vi "Open Utility Motors.vi"(9 "CAN IDs":u8[](array[numeric])=[0, 0, 0, 0, 0, 0, 0]) -> ()   [LabVIEW 2018]
uses:
  <vilib>/Rock Robotics/WPI/ThirdParty/Phoenix-LabVIEW/Motor Controller/Controls/CTRE_Phoenix_MotorControl_NeutralMode.ctl
  <vilib>/Rock Robotics/WPI/Switch/WPI_SwitchOpenLimit.vi
  <vilib>/Rock Robotics/SystemInterfaces/DIO/FPGA_DIOChannel.ctl
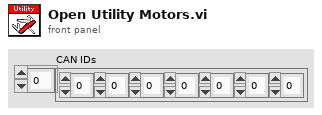
[diagram p1: front panel]
types:
  T1 = typedef "CTRE_Phoenix_MotorControl_NeutralMode.ctl" = enum8{"EEPROMSetting", "Override to Coast", "Override to Brake"}
  T2 = typedef "WPI_MotorControlDeviceRef.ctl" = cluster{"DeviceStatus":errorcluster, "Type":T3, "PWM":cluster{"PWM Channel":T4, "DeadBand":T5}, "CAN":cluster{"Device Number":u8, "SetOutput VI Ref":variant, "GetOutput VI Ref":variant, "Enable VI Ref":variant, "Disable VI Ref":variant, "Data":variant}, "Invert":bool, "DIO PWM":cluster{"PWM \"Enable\" Channel":T4, "DIOChannel":T6, "PWM Rate":dbl}}
  T3 = typedef "WPI_MotorControlType.ctl" = enum16{"PWM", "CAN", "DIO PWM"}
  T4 = typedef "FPGA_DIOPWMChannel.ctl" = enum8{"PWM 0", "PWM 1", "PWM 2", "PWM 3", "PWM 4", "PWM 5", "PWM 6", "PWM 7", "PWM 8", "PWM 9", "PWM MXP 0", "PWM MXP 1", "PWM MXP 2", "PWM MXP 3", "PWM MXP 4", "PWM MXP 5", "PWM MXP 6", "PWM MXP 7", "PWM MXP 8", "PWM MXP 9", "Invalid"}
  T5 = typedef "WPI_PWMDeadband.ctl" = cluster{"Name":string, "maxPositivePwm":i32, "minPositivePwm":i32, "centerPwm":i32, "maxNegativePwm":i32, "minNegativePwm":i32, "angularRange":u16}
  T6 = typedef "FPGA_DIOChannel.ctl" = enum8{"DIO 0", "DIO 1", "DIO 2", "DIO 3", "DIO 4", "DIO 5", "DIO 6", "DIO 7", "DIO 8", "DIO 9", "DIO MXP 0", "DIO MXP 1", "DIO MXP 2", "DIO MXP 3", "DIO MXP 4", "DIO MXP 5", "DIO MXP 6", "DIO MXP 7", "DIO MXP 8", "DIO MXP 9", "DIO MXP 10", "DIO MXP 11", "DIO MXP 12", "DIO MXP 13", "DIO MXP 14", "DIO MXP 15", "SPI Port CS1", "SPI Port CS2", "SPI Port CS3", "SPI Port MISO", "SPI Port MOSI", "Invalid"}
  T7 = typedef "WPI_SwitchDevRef.ctl" = cluster{"DevStatus":errorcluster, "DIO Channel":T6, "CntIndex":T8, "Normally Closed":bool}
  T8 = typedef "FPGA_CounterCtrSystemIndex.ctl" = enum8{"Ctr 0", "Ctr 1", "Ctr 2", "Ctr 3", "Ctr 4", "Ctr 5", "Ctr 6", "Ctr 7", "Invalid"}
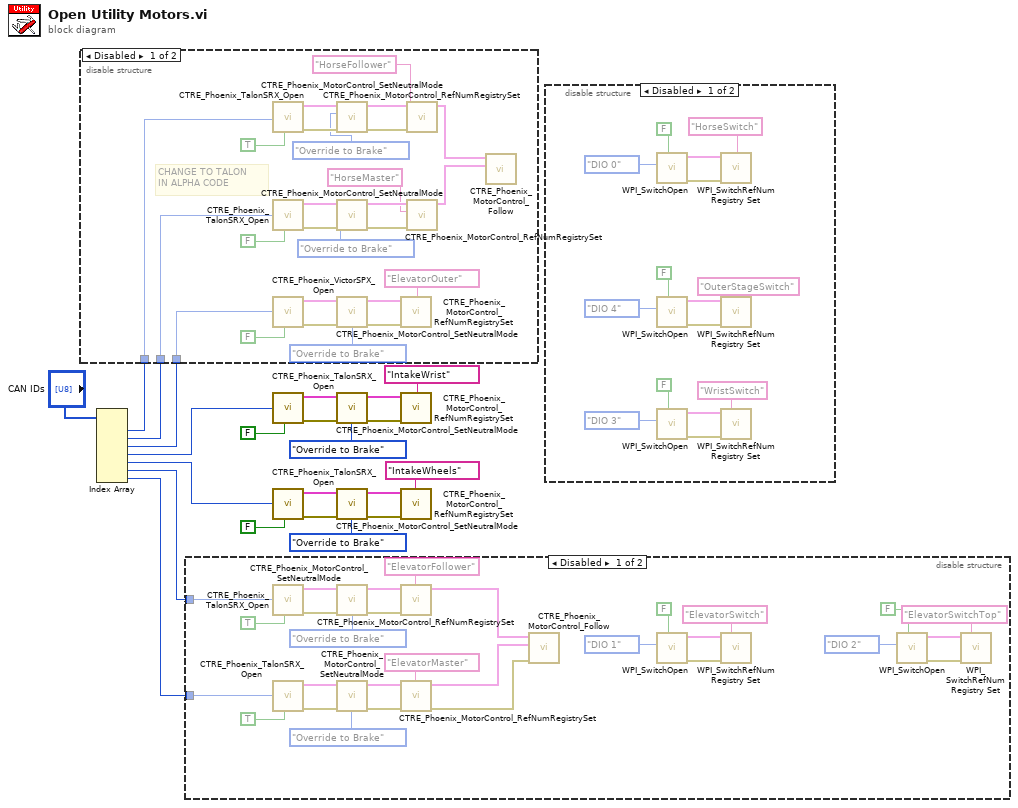
[diagram p0: block diagram]
diagram:
  n1 = Index Array(array="CAN IDs") -> (element #1=w8:u8, element #2=w7:u8, element #3=w6:u8, element #4=w5:u8, element #5=w4:u8, element #6=w3:u8, element #7=w2:u8)  [unwired: 7 in]
  n2 = disable-structure shown="Disabled" {
    disable-tunnel: w8 -> [w39 _]
    disable-tunnel: w7 -> [w38 _]
    disable-tunnel: w6 -> [w37 _]
    frame Disabled {
      # "CHANGE TO TALON\nIN ALPHA CODE"
      n3 = call <vilib>:"CTRE_Phoenix_TalonSRX_Open.vi"("Invert"=TRUE, "Device Number"=w39) -> ("error out"=w30:errorcluster, "CAN Talon SRX Ref"=w32:T2)  [unwired: 8 in]
      n4 = call <vilib>:"CTRE_Phoenix_TalonSRX_Open.vi"("Invert"=FALSE, "Device Number"=w38) -> ("error out"=w34:errorcluster, "CAN Talon SRX Ref"=w36:T2)  [unwired: 8 in]
      n5 = call <vilib>:"CTRE_Phoenix_VictorSPX_Open.vi"("Invert"=FALSE, "Device Number"=w37) -> ("error out"=w48:errorcluster, "CAN Talon SRX Ref"=w46:T2)  [unwired: 8 in]
      n6 = call <vilib>:"CTRE_Phoenix_MotorControl_SetNeutralMode.vi"("error in (no error)"=w30, "Motor Control Neutral Mode"=CTRE_Phoenix_MotorControl_NeutralMode."Override to Brake", "PhoenixMotorControlDevRef"=w32) -> ("error out"=w29:errorcluster, "PhoenixMotorControlDevRef"=w31:T2)  [unwired: 7 in]
      n7 = call <vilib>:"CTRE_Phoenix_MotorControl_SetNeutralMode.vi"("error in (no error)"=w34, "Motor Control Neutral Mode"=CTRE_Phoenix_MotorControl_NeutralMode."Override to Brake", "PhoenixMotorControlDevRef"=w36) -> ("error out"=w33:errorcluster, "PhoenixMotorControlDevRef"=w35:T2)  [unwired: 7 in]
      n8 = call <vilib>:"CTRE_Phoenix_MotorControl_SetNeutralMode.vi"("error in (no error)"=w48, "Motor Control Neutral Mode"=CTRE_Phoenix_MotorControl_NeutralMode."Override to Brake", "PhoenixMotorControlDevRef"=w46) -> ("error out"=w47:errorcluster, "PhoenixMotorControlDevRef"=w45:T2)  [unwired: 7 in]
      n9 = call <vilib>:"CTRE_Phoenix_MotorControl_RefNumRegistrySet.vi"("error in (no error)"=w47, "refnum name"="ElevatorOuter", "PhoenixMotorControlDevRef"=w45) -> ()  [unwired: 7 in, 2 out]
      n10 = call <vilib>:"CTRE_Phoenix_MotorControl_RefNumRegistrySet.vi"("error in (no error)"=w29, "refnum name"="HorseFollower", "PhoenixMotorControlDevRef"=w31) -> ("PhoenixMotorControlDevRef"=w28:T2)  [unwired: 7 in, 1 out]
      n11 = call <vilib>:"CTRE_Phoenix_MotorControl_RefNumRegistrySet.vi"("error in (no error)"=w33, "refnum name"="HorseMaster", "PhoenixMotorControlDevRef"=w35) -> ("PhoenixMotorControlDevRef"=w27:T2)  [unwired: 7 in, 1 out]
      n12 = call <vilib>:"CTRE_Phoenix_MotorControl_Follow.vi"("Master Controller to Follow"=w27, "PhoenixMotorControlDevRef"=w28) -> ()  [unwired: 8 in, 2 out]
    }
    frame Enabled {
    }
  }
  n13 = disable-structure shown="Disabled" {
    disable-tunnel: w3 -> [w63 _]
    disable-tunnel: w2 -> [w62 _]
    frame Disabled {
      n14 = call <vilib>:"CTRE_Phoenix_TalonSRX_Open.vi"("Invert"=TRUE, "Device Number"=w63) -> ("error out"=w77:errorcluster, "CAN Talon SRX Ref"=w73:T2)  [unwired: 8 in]
      n15 = call <vilib>:"CTRE_Phoenix_TalonSRX_Open.vi"("Invert"=TRUE, "Device Number"=w62) -> ("error out"=w75:errorcluster, "CAN Talon SRX Ref"=w71:T2)  [unwired: 8 in]
      n16 = call <vilib>:"CTRE_Phoenix_MotorControl_SetNeutralMode.vi"("error in (no error)"=w77, "Motor Control Neutral Mode"=CTRE_Phoenix_MotorControl_NeutralMode."Override to Brake", "PhoenixMotorControlDevRef"=w73) -> ("error out"=w76:errorcluster, "PhoenixMotorControlDevRef"=w72:T2)  [unwired: 7 in]
      n17 = call <vilib>:"CTRE_Phoenix_MotorControl_SetNeutralMode.vi"("error in (no error)"=w75, "Motor Control Neutral Mode"=CTRE_Phoenix_MotorControl_NeutralMode."Override to Brake", "PhoenixMotorControlDevRef"=w71) -> ("error out"=w74:errorcluster, "PhoenixMotorControlDevRef"=w70:T2)  [unwired: 7 in]
      n18 = call <vilib>:"CTRE_Phoenix_MotorControl_RefNumRegistrySet.vi"("error in (no error)"=w76, "refnum name"="ElevatorFollower", "PhoenixMotorControlDevRef"=w72) -> ("PhoenixMotorControlDevRef"=w61:T2)  [unwired: 7 in, 1 out]
      n19 = call <vilib>:"CTRE_Phoenix_MotorControl_RefNumRegistrySet.vi"("error in (no error)"=w74, "refnum name"="ElevatorMaster", "PhoenixMotorControlDevRef"=w70) -> ("error out"=w59:errorcluster, "PhoenixMotorControlDevRef"=w60:T2)  [unwired: 7 in]
      n20 = call <vilib>:"CTRE_Phoenix_MotorControl_Follow.vi"("error in (no error)"=w59, "Master Controller to Follow"=w60, "PhoenixMotorControlDevRef"=w61) -> ()  [unwired: 7 in, 2 out]
      n21 = call-poly <vilib>:"WPI_SwitchOpen.vi"("Normally Closed"=FALSE, "DIO Channel"=FPGA_DIOChannel."DIO 1") -> ("error out"=w57:errorcluster, "SwitchDevRef"=w56:T7)  [unwired: 8 in]
      n22 = call <vilib>:"WPI_SwitchRefNum Registry Set.vi"("error in (no error)"=w57, "refnum name"="ElevatorSwitch", "SwitchDevRef"=w56) -> ()  [unwired: 7 in, 2 out]
      n23 = call-poly <vilib>:"WPI_SwitchOpen.vi"("Normally Closed"=FALSE, "DIO Channel"=FPGA_DIOChannel."DIO 2") -> ("error out"=w50:errorcluster, "SwitchDevRef"=w51:T7)  [unwired: 8 in]
      n24 = call <vilib>:"WPI_SwitchRefNum Registry Set.vi"("error in (no error)"=w50, "refnum name"="ElevatorSwitchTop", "SwitchDevRef"=w51) -> ()  [unwired: 7 in, 2 out]
    }
    frame Enabled {
    }
  }
  n25 = call <vilib>:"CTRE_Phoenix_TalonSRX_Open.vi"("Invert"=FALSE, "Device Number"=w5) -> ("error out"=w22:errorcluster, "CAN Talon SRX Ref"=w18:T2)  [unwired: 8 in]
  n26 = call <vilib>:"CTRE_Phoenix_TalonSRX_Open.vi"("Invert"=FALSE, "Device Number"=w4) -> ("error out"=w20:errorcluster, "CAN Talon SRX Ref"=w16:T2)  [unwired: 8 in]
  n27 = call <vilib>:"CTRE_Phoenix_MotorControl_SetNeutralMode.vi"("error in (no error)"=w22, "Motor Control Neutral Mode"=CTRE_Phoenix_MotorControl_NeutralMode."Override to Brake", "PhoenixMotorControlDevRef"=w18) -> ("error out"=w21:errorcluster, "PhoenixMotorControlDevRef"=w17:T2)  [unwired: 7 in]
  n28 = call <vilib>:"CTRE_Phoenix_MotorControl_SetNeutralMode.vi"("error in (no error)"=w20, "Motor Control Neutral Mode"=CTRE_Phoenix_MotorControl_NeutralMode."Override to Brake", "PhoenixMotorControlDevRef"=w16) -> ("error out"=w19:errorcluster, "PhoenixMotorControlDevRef"=w15:T2)  [unwired: 7 in]
  n29 = call <vilib>:"CTRE_Phoenix_MotorControl_RefNumRegistrySet.vi"("error in (no error)"=w21, "refnum name"="IntakeWrist", "PhoenixMotorControlDevRef"=w17) -> ()  [unwired: 7 in, 2 out]
  n30 = call <vilib>:"CTRE_Phoenix_MotorControl_RefNumRegistrySet.vi"("error in (no error)"=w19, "refnum name"="IntakeWheels", "PhoenixMotorControlDevRef"=w15) -> ()  [unwired: 7 in, 2 out]
  n31 = disable-structure shown="Disabled" {
    frame Disabled {
      n32 = call-poly <vilib>:"WPI_SwitchOpen.vi"("Normally Closed"=FALSE, "DIO Channel"=FPGA_DIOChannel."DIO 0") -> ("error out"=w91:errorcluster, "SwitchDevRef"=w92:T7)  [unwired: 8 in]
      n33 = call-poly <vilib>:"WPI_SwitchOpen.vi"("Normally Closed"=FALSE, "DIO Channel"=FPGA_DIOChannel."DIO 4") -> ("error out"=w81:errorcluster, "SwitchDevRef"=w80:T7)  [unwired: 8 in]
      n34 = call-poly <vilib>:"WPI_SwitchOpen.vi"("Normally Closed"=FALSE, "DIO Channel"=FPGA_DIOChannel."DIO 3") -> ("error out"=w84:errorcluster, "SwitchDevRef"=w85:T7)  [unwired: 8 in]
      n35 = call <vilib>:"WPI_SwitchRefNum Registry Set.vi"("error in (no error)"=w91, "refnum name"="HorseSwitch", "SwitchDevRef"=w92) -> ()  [unwired: 7 in, 2 out]
      n36 = call <vilib>:"WPI_SwitchRefNum Registry Set.vi"("error in (no error)"=w81, "refnum name"="OuterStageSwitch", "SwitchDevRef"=w80) -> ()  [unwired: 7 in, 2 out]
      n37 = call <vilib>:"WPI_SwitchRefNum Registry Set.vi"("error in (no error)"=w84, "refnum name"="WristSwitch", "SwitchDevRef"=w85) -> ()  [unwired: 7 in, 2 out]
    }
    frame Enabled {
    }
  }
